vi "AVS_Activate.vi"(7 "a_pDeviceId":u8[](array[numeric])) -> (4 "Output Value":i32, 8 "a_pDeviceId":u8[](array[numeric]))   [LabVIEW 2013, in "Avantes Spectrometer Functions.lvlib"]
uses:
  Avantes Spectrometer Functions.lvlib
  AvantesSpectrometer2/polling_mc/AS5216.dll
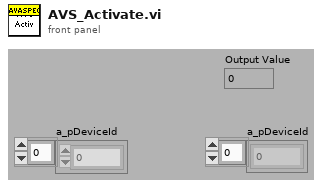
[diagram p1: front panel]
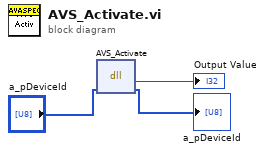
[diagram p0: block diagram]
diagram:
  n1 = dll-call lib="C:/Users/dhstuart/Dropbox/CLTC/AvantesSpectrometer2/polling_mc/AS5216.dll" fn="AVS_Activate"("a_pDeviceId"="a_pDeviceId") -> (→"Output Value":i32, "a_pDeviceId"=→"a_pDeviceId":u8[])  [unwired: 3 in, 2 out]
